vi "Camera.UnInit.vi"(8 "error in (no error)":errorcluster, 11 "Camera.Simulated":refnum<class "Camera.IMAQdx.lvclass">) -> (0 "error out":errorcluster, 3 "Camera.Simulated out":refnum<class "Camera.IMAQdx.lvclass">)   [LabVIEW 2020, in "Camera.IMAQdx.lvclass"]
doc: "---------------------------------------------------------------\nJKI State Machine Objects™\nhttp://jki.net/state-machine-objects/\nCopyright (C) 2005-2015, JKI <info@jki.net>\nALL RIGHTS RESERVEDJKI State Machine Objects (SMO) 1.0.0.5\nJKI - JKI\nCopyright (c) 2016, JKI"
uses:
  Camera.IMAQdx.lvclass
  Camera.IMAQdx.lvclass/Camera.IMAQdx.ctl
  Camera/Camera.lvclass
  <vilib>/vision/driver/NI_Vision_Acquisition_Software.lvlib
panel:
  # "For instructions on how to use the JKI State Machine Objects, examples and video tutorials, visit:\nhttp://jki.net/state-machine-objects/\n\nJKI State Machine Objects™\nhttp://jki.net/state-machine-objects/\nCopyright (C) 2005-2015, JKI <info@jki.net>\nALL RIGHTS RESERVED"
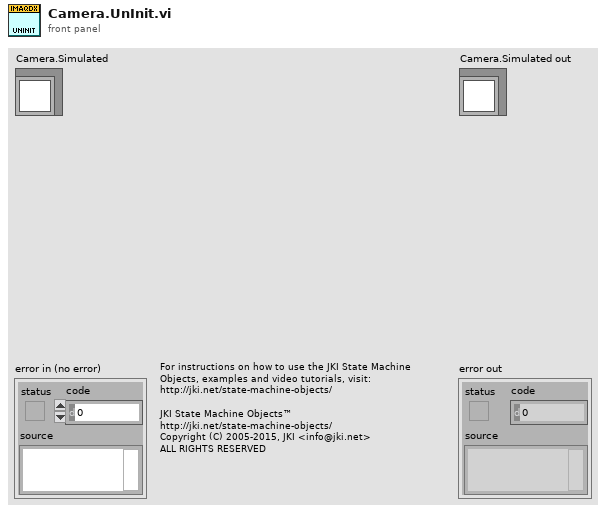
[diagram p1: front panel]
types:
  T1 = typedef "IMAQ Image.ctl" = refnum<image>
  T2 = typedef "IMAQdx.ctl" = refnum<k21>
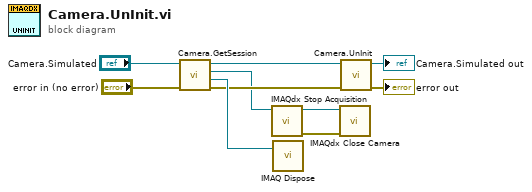
[diagram p0: block diagram]
diagram:
  n1 = call "Camera.GetSession.vi"("error in (no error)"="error in (no error)", "Camera.Simulated"="Camera.Simulated") -> ("error out"=w4:errorcluster, "Image"=w8:T1, "Session"=w2:T2, "Camera.Simulated"=w6:refnum<class "Camera.IMAQdx.lvclass">)  [unwired: 6 in]
  n2 = call <vilib>:"IMAQdx Stop Acquisition.vi"("Session In"=w2) -> ("error out"=w1:errorcluster, "Session Out"=w3:T2)  [unwired: 9 in]
  n3 = call "IMAQ Dispose"("Image"=w8) -> ()  [unwired: 5 in, 1 out]
  n4 = call <vilib>:"IMAQdx Close Camera.vi"("error in"=w1, "Session In"=w3) -> ()  [unwired: 9 in, 1 out]
  n5 = call-parent "Camera.UnInit.vi"("error in (no error)"=w4, "Camera"=w6) -> ("error out"=→"error out":errorcluster, "Camera out"=→"Camera.Simulated out":refnum<class "Camera.IMAQdx.lvclass">)  [unwired: 8 in]
